vi "Subscribe Actor to Topic.vi"(4 "Excluded (None)":refnum<class "Message.lvclass">[](array[class]), 5 "Channel Class":refnum<class "Pub Sub Message Channel.lvclass">, 6 "Included (All)":refnum<class "Message.lvclass">[](array[class]), 8 "error in (no error)":errorcluster, 9 "Name":string, 10 "Receivers Enqueuer":refnum<class "Message Enqueuer.lvclass">, 11 "Topic":string) -> (0 "error out":errorcluster, 2 "New Subscription":bool, 3 "Channel Out":refnum<class "Pub Sub Message Channel.lvclass">)   [LabVIEW 2020, in "Actor Pub Sub Channels.lvlib"]
uses:
  Actor Pub Sub Channels.lvlib
  <vilib>/ActorFramework/Message Enqueuer/Message Enqueuer.lvclass
  Pub Sub Message Channel/Pub Sub Message Channel.lvclass
  <vilib>/ActorFramework/Message/Message.lvclass
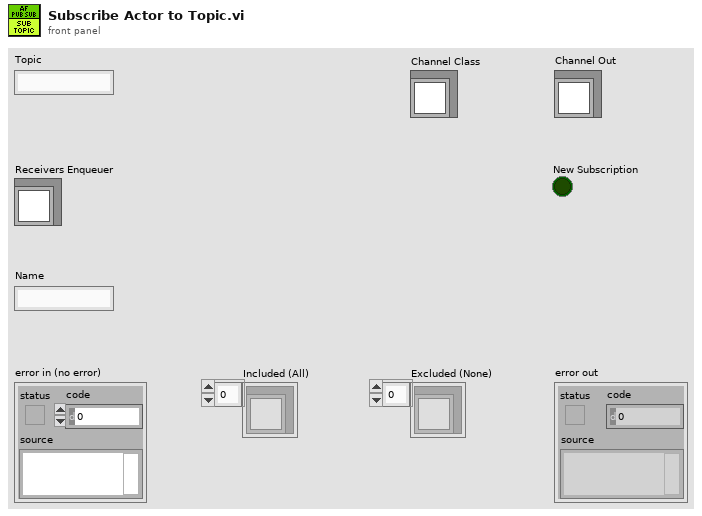
[diagram p1: front panel]
types:
  T1 = enum16{"Nothing", "Get Channel", "Get Or Create Channel", "Close Channel", "Dispose"}
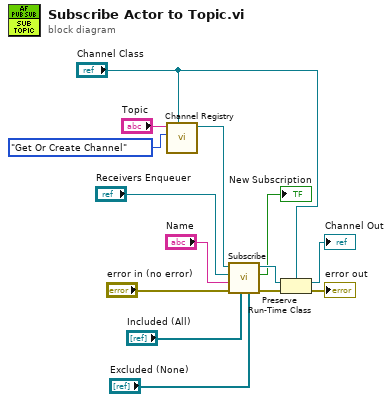
[diagram p0: block diagram]
diagram:
  n1 = call "Channel Registry.vi"("New Channel Class"="Channel Class", "Action"=T1."Get Or Create Channel", "Topic"="Topic") -> ("Pub Sub Message Channel"=w12:refnum<class "Pub Sub Message Channel.lvclass">)  [unwired: 6 in, 2 out]
  n2 = call-dynamic "Subscribe.vi"("Excluded (None)"="Excluded (None)", "Included (All)"="Included (All)", "error in (no error)"="error in (no error)", "Name"="Name", "Receivers Enqueuer"="Receivers Enqueuer", "Pub Sub Message Channel in"=w12) -> ("error out"=w9:errorcluster, "New Subscription"=→"New Subscription":bool, "Pub Sub Message Channel out"=w7:refnum<class "Pub Sub Message Channel.lvclass">)  [unwired: 3 in]
  n3 = Preserve Run-Time Class(object in=w7, error in=w9, 2:"Channel Class") -> (object out=→"Channel Out":refnum<class "Pub Sub Message Channel.lvclass">, error out=→"error out":errorcluster)
